vi "Create Audio Spectrum (SubVI).vi"(9 "Sample Period (ms)":dbl, 10 "Raw Audio":i16[](array[numeric]), 11 "Filtered Audio":dbl[](array[numeric])) -> (3 "FFT Out":dynamicdata(waveform))   [LabVIEW 2021]
uses:
  <vilib>/express/express analysis/Spectral/Block/exnSpectralBlock spectral measurements power poly.vi
  <vilib>/express/express analysis/Spectral/Block/exnSpectralBlock spectral measurements power DDT.vi
  <vilib>/express/express analysis/Spectral/XNode/ExpressSpectralMeasurementsBlockNode.xnode
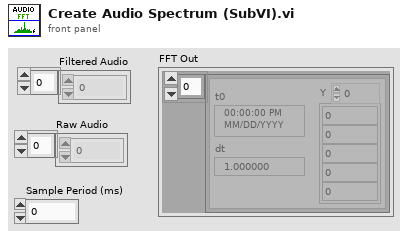
[diagram p1: front panel]
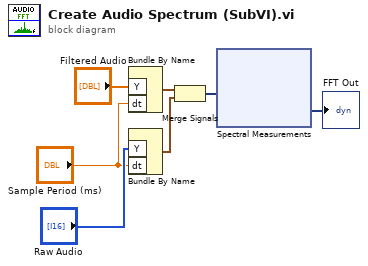
[diagram p0: block diagram]
diagram:
  n1 = Bundle By Name("Y"="Filtered Audio", "dt"="Sample Period (ms)") -> (w4:waveform(dbl))  [unwired: 1 in]
  n2 = Bundle By Name("Y"="Raw Audio", "dt"="Sample Period (ms)") -> (w1:waveform(i16))  [unwired: 1 in]
  n3 = Merge Signals(w4, w1) -> (w2:dynamicdata)
  n4 = xnode ("Spectral Measurements")("Signals"=w2) -> ("Power Spectrum"=→"FFT Out":dynamicdata)  [unwired: 2 in, 2 out]
